vi "Get print offset.vi"(8 "error in (no error)":errorcluster, 11 "Domino Laser module Class in":refnum<class "Domino Laser module Class.lvclass">) -> (0 "error out":errorcluster, 3 "Domino Laser module Class out":refnum<class "Domino Laser module Class.lvclass">)   [LabVIEW 2015, in "Domino LM.lvlib" / "Domino Laser module Class.lvclass"]
uses:
  CTRLS/Domino Laser module Class.lvclass
  CTRLS/Domino Laser module Class.lvclass/Domino Laser module Class.ctl
panel:
  out "X offset":string
  out "Y offset":string
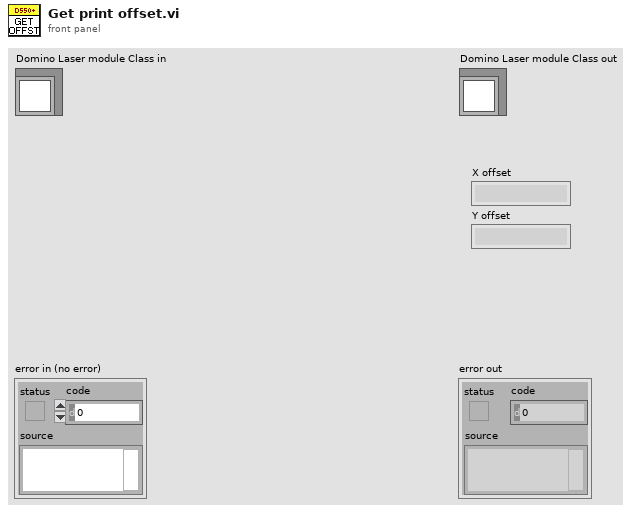
[diagram p1: front panel]
types:
  T1 = cluster{"Camera Offset [MM]":u32, "Reject Offset [MM]":u32, "Reject Delay [% of Width]":u32, "Carton Width [MM]":u32, "Carton Width Error [MM] ":u16, "Reject Verify Offset [MM]":u32, "Gate Width B [MM] \n":u32, "Printer offset X":i16, "Printer offset Y":i16}
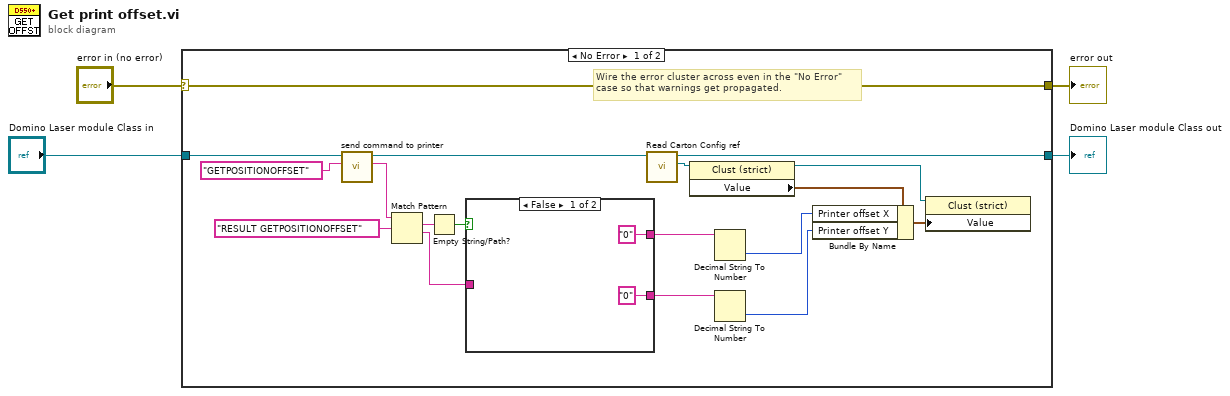
[diagram p0: block diagram]
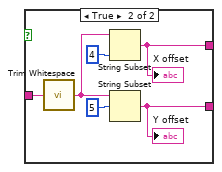
[diagram p2: hidden frame]
diagram:
  n1 = case shown="No Error" "error in (no error)" {
    selector: "error in (no error)" -> [w22 w32]
    tunnel: [w22 w32] -> w3
    tunnel: [w11 w31] -> w1
    tunnel: "Domino Laser module Class in" -> [w17 w31]
    frame No Error {
      # "Wire the error cluster across even in the \"No Error\"\ncase so that warnings get propagated."
      n2 = call "send command to printer.vi"("command to be sent"="GETPOSITIONOFFSET", "Domino Laser module Class in"=w17) -> ("Recived message"=w15:string, "Domino Laser module Class out"=w12:refnum<class "Domino Laser module Class.lvclass">)  [unwired: 6 in, 2 out]
      n3 = Match Pattern(string=w15, regular expression="RESULT GETPOSITIONOFFSET") -> (match substring=w18:string, after substring=w20:string)  [unwired: 1 in, 2 out]
      n4 = Empty String/Path?(string/path=w18) -> (empty?=w19:bool)
      n5 = case shown="False" w19 {
        tunnel: w20 -> [_ w27]
        tunnel: ["0" ("trimmed string") w26] -> w14
        tunnel: ["0" ("trimmed string") w25] -> w13
        frame False {
        }
        frame True {
          n6 = call <vilib>:"Trim Whitespace.vi"("string"=w27) -> ("trimmed string"=w29:string)  [unwired: 1 in]
          n7 = String Subset(string=w29, length (rest)=4 ("length (rest)")) -> (substring=w25:string)  [unwired: 1 in]
          "X offset" <- w25
          n8 = String Subset(string=w29, offset (0)=5) -> (substring=w26:string)  [unwired: 1 in]
          "Y offset" <- w26
        }
      }
      n9 = call "Read Carton Config ref.vi"("Domino Laser module Class in"=w12) -> ("Carton Config"=w10:refnum<vi>, "Domino Laser module Class out"=w11:refnum<class "Domino Laser module Class.lvclass">)  [unwired: 8 in, 1 out]
      n10 = property class="Clust (strict)"(reference=w10) -> (reference out=w5:refnum<vi>, "Value"=w9:T1)  [unwired: 1 in, 1 out]
      n11 = Decimal String To Number(string=w13) -> (number=w8:i32)  [unwired: 2 in, 1 out]
      n12 = Decimal String To Number(string=w14) -> (number=w7:i32)  [unwired: 2 in, 1 out]
      n13 = Bundle By Name(cluster=w9, "Printer offset X"=w8, "Printer offset Y"=w7) -> (w6:T1)
      n14 = property class="Clust (strict)"(reference=w5, "Value"=w6) -> ()  [unwired: 1 in, 2 out]
    }
    frame Error {
    }
  }
  "error out" <- w3
  "Domino Laser module Class out" <- w1
